vi "SEND_RTC_TIME.vi"(8 "error in (no error)":errorcluster, 11 "Message":T2={"Payload Size"=0, "Sequence Number"=0, "Sensor Type"=enum."APP", "Message Types"=enum."SEND_LOG_FILE_SIZE", "Data"=[]}) -> (0 "error out":errorcluster, 3 "Current RTC Time":T1)   [LabVIEW 2019]
uses:
  Typedefs/Message.ctl
  Typedefs/Sensor Types.ctl
  Typedefs/Message Types.ctl
  <vilib>/Utility/miscctls.llb/LVDateTimeRec.ctl
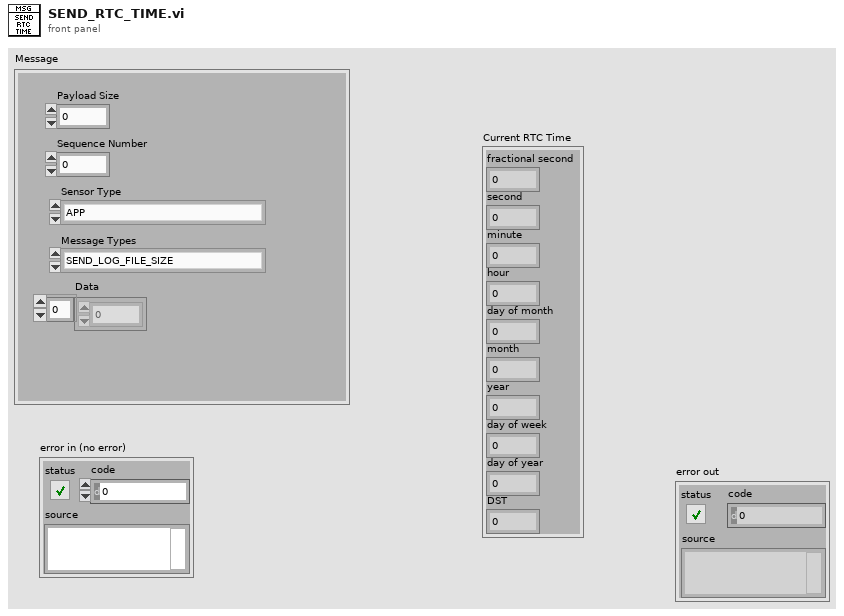
[diagram p1: front panel]
types:
  T1 = typedef "LVDateTimeRec.ctl" = cluster{"fractional second":dbl, "second":i32, "minute":i32, "hour":i32, "day of month":i32, "month":i32, "year":i32, "day of week":i32, "day of year":i32, "DST":i32}
  T2 = typedef "Message.ctl" = cluster{"Payload Size":u8, "Sequence Number":u8, "Sensor Type":T3, "Message Types":T4, "Data":u8[]}
  T3 = typedef "Sensor Types.ctl" = enum16{"APP", "TURBIDITY", "PH"}
  T4 = typedef "Message Types.ctl" = enum16{"HEART_BEAT", "CONNECT", "GET_CURRENT_MEASUREMENTS", "GET_LOG_FILE", "SEND_LOG_FILE_SIZE", "SEND_LOG_FILE_CHUNK", "GET_LOGGING_PERIOD", "SET_LOGGING_PERIOD", "SEND_SD_CARD_INFO", "GET_LOGS_LIST", "SEND_LOG_FILE_NAME", "SEND_LOGGING_PERIOD", "GET_RTC_TIME", "SET_RTC_TIME", "SEND_RTC_TIME", "SEND_CURRENT_MEASUREMENTS", "DELETE_LOG_FILE", "GET_SD_CARD_INFO", "GET_BATTERY_INFO", "SEND_BATTERY_INFO", "GET_LOG_FILE_SIZE", "ERROR_MSG"}
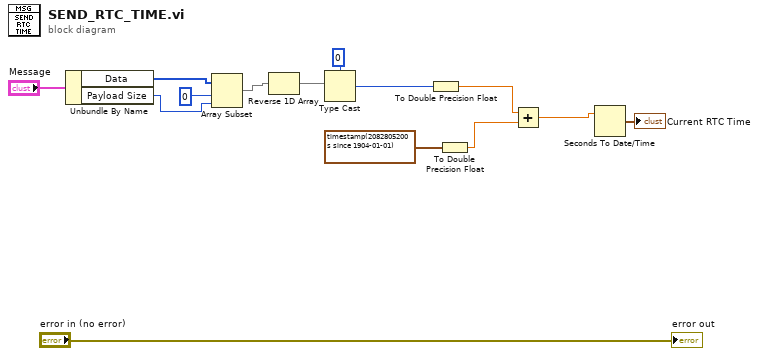
[diagram p0: block diagram]
diagram:
  n1 = Unbundle By Name("Message") -> ("Data"=w2:u8[], "Payload Size"=w1:u8)
  n2 = Array Subset(array=w2, index=0, length=w1) -> (w11:u8[])
  n3 = Reverse 1D Array(array=w11) -> (reversed array=w10:u8[])
  n4 = Type Cast(type=u32 0, x=w10) -> (*(type *) &x=w8:u32)
  n5 = To Double Precision Float(number=w8) -> (double precision float=w7:dbl)
  n6 = To Double Precision Float(number=timestamp(2082805200 s since 1904-01-01)) -> (double precision float=w6:dbl)
  n7 = Add(x=w7, y=w6) -> (x+y=w5:dbl)
  n8 = Seconds To Date/Time(time stamp (now)=w5) -> (date time rec=→"Current RTC Time":T1)  [unwired: 1 in]
  "error out" <- "error in (no error)"
